vi "SmartSEM Remote API set string.vi"(5 "Wait (ms)":u32, 7 "Iterations":u32=3, 8 "error in":errorcluster, 9 "vValue":string, 10 "lpszParam":string, 11 "Api":refnum<k7>(container)) -> (0 "error out":errorcluster, 3 "Api out":refnum<k7>)   [LabVIEW 2018]
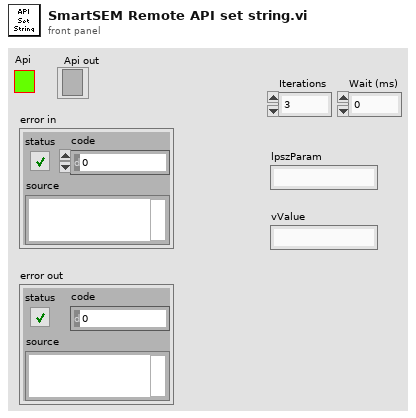
[diagram p1: front panel]
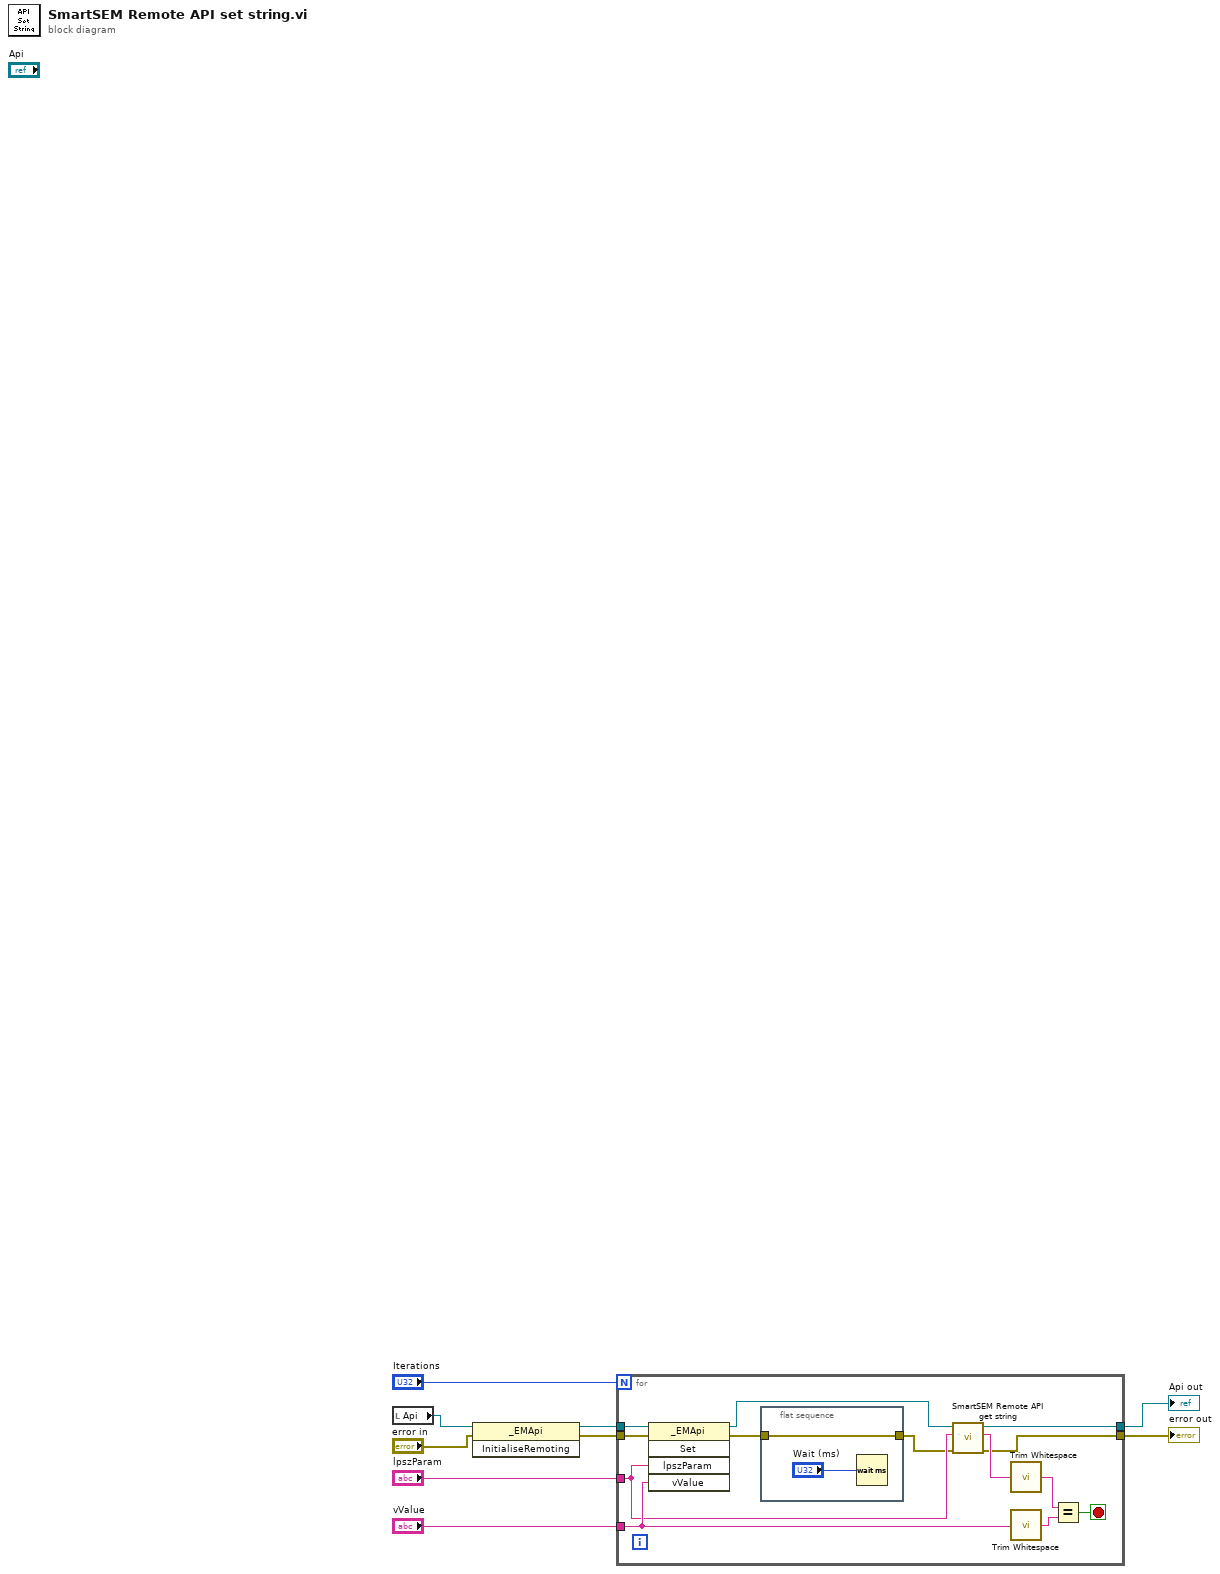
[diagram p0: block diagram]
diagram:
  n1 = local read "Api"() -> (w9:refnum<k7>)
  n2 = invoke class="_EMApi" method="InitialiseRemoting"(reference=w9, error in="error in") -> (reference out=w8:refnum<k7>, error out=w7:errorcluster)  [unwired: 1 in, 1 out]
  n3 = for {
    N: "Iterations" -> [_]
    tunnel: w8 -> [w22]
    tunnel: w7 -> [w21]
    tunnel: [w12] -> w2
    tunnel: [w11] -> w1
    tunnel: "vValue" -> [w18]
    tunnel: "lpszParam" -> [w14]
    stop <- w19 stop-if-true
    n4 = invoke class="_EMApi" method="Set"(reference=w22, error in=w21, "lpszParam"=w14, "vValue"=w18) -> (reference out=w15:refnum<k7>, error out=w16:errorcluster)  [unwired: 1 in, 3 out]
    n5 = flat-sequence {
      tunnel: [w24] -> w10
      tunnel: w16 -> [w24]
      frame #0 {
        n6 = Wait (ms)(milliseconds to wait="Wait (ms)") -> ()  [unwired: 1 out]
      }
    }
    n7 = call "SmartSEM Remote API get string.vi"("error in"=w10, "lpszParam"=w14, "Api"=w15) -> ("error out"=w11:errorcluster, "data"=w13:string, "Api out"=w12:refnum<k7>)  [unwired: 6 in]
    n8 = call <vilib>:"Trim Whitespace.vi"("string"=w13) -> ("trimmed string"=w20:string)  [unwired: 1 in]
    n9 = call <vilib>:"Trim Whitespace.vi"("string"=w18) -> ("trimmed string"=w17:string)  [unwired: 1 in]
    n10 = Equal?(x=w20, y=w17) -> (x = y?=w19:bool)
  }
  "Api out" <- w2
  "error out" <- w1
